vi "MagnetometerStateMachine-LakeshoreGaussMeter.vi"() -> ()   [LabVIEW 2014]
uses:
  <vilib>/MakerHub/LINX/Private/Local IO/LinxI2cWrite.vi
  <vilib>/MakerHub/LINX/Public/Utilities/Check Channel.vi
  <vilib>/MakerHub/LINX/Public/Utilities/Open Serial.vi
  <vilib>/MakerHub/LINX/Private/Utilties/Generate Error.vi
  <instrlib>/Stanford Research 830/Public/Data/Read (All Parameters).vi
  <vilib>/express/express shared/transition.llb/Dynamic To Waveform Array.vi
  <vilib>/express/express signal manip/GetorSetDDTAttributes/Get DDT Attributes/Get DDT Properties.xnode
  <vilib>/MakerHub/LINX/LMH-LINX.lvlib
  <instrlib>/Stanford Research 830/Stanford Research 830.lvlib
panel:
  out "data array":T1(array[cluster])
  in  "delta DAC":dbl=0.01 min=0.0 max=1.0 step=0.001 format="%#_13g"
  in  "max DAC":sgl=4.0 min=0 max=5 step=0.001
  in  "min DAC":dbl=1.0 min=0.0 max=5.0 step=0.001 format="%#_13g"
  out "Nloops2":i32
  out "Nloops":i32
  out "SRS-T":dbl
  out "SRS-R":dbl
  out "SRS-Y":dbl
  out "Parameter Values":T2
  out "XY Graph":T3(graph)
  out "SRS-X":dbl
  in  "Time Constant (8: 100ms)":u16(ring)=8 items=["10 us", "30 us", "100 us", "300 us", "1 ms", "3 ms", "10 ms", "30 ms", "100 ms", "300 ms", "1 s", "3 s", "10 s", "30 s", "100 s", "300 s", "1 ks", "3 ks", "10 ks", "30 ks"]
  in  "Internal Reference Frequency (1000 Hz)":dbl=20.0
  in  "Sine Output Amplitude (1 V)":dbl=1.0
  in  "Sensitivity (26: 1 V/uA)":i16(ring)=26 items=["Auto Gain"=-1, "2 nV/fA"=0, "5 nV/fA"=1, "10 nV/fA"=2, "20 nV/fA"=3, "50 nV/fA"=4, "100 nV/fA"=5, "200 nV/fA"=6, "500 nV/fA"=7, "1 uV/pA"=8, "2 uV/pA"=9, "5 uV/pA"=10, "10 uV/pA"=11, "20 uV/pA"=12, "50 uV/pA"=13, "100 uV/pA"=14, "200 uV/pA"=15, "500 uV/pA"=16, "1 mV/nA"=17, "2 mV/nA"=18, "5 mV/nA"=19, "10 mV/nA"=20, "20 mV/nA"=21, "50 mV/nA"=22, "100 mV/nA"=23, "200 mV/nA"=24, "500 mV/mA"=25, "1 V/uA"=26]
  in  "Dynamic Reserve (2: Low Noise)":i16(ring)=2 items=["High Reserve"=0, "Normal"=1, "Low Noise"=2, "Auto Reserve"=-1]
  in  "Reference Source (1: Internal)":u16(ring)=1 items=["External", "Internal"]
  in  "Input Coupling (0: AC)":u16(ring) items=["AC", "DC"]
  in  "Input Connection (0: Single-Ended Voltage)":u16(ring) items=["Single-Ended Voltage", "Differential Voltage", "1 MOhm Current Gain", "100 MOhm Current Gain"]
  in  "Current DAC Value":dbl
  in  "DAC Zeroing Voltage":dbl=2.5 min=0.0 max=5.0 step=0.001 format="%#_6f"
  out "Magnetic Field (Oe)":dbl
  in  "Choices":T4(ring)
  in  "End It All!":bool
  out "Error Out":errorcluster={"status"=FALSE, "code"=1073676294, "source"="VISA Read in LVH-LINX.lvlib:Device.lvlib:Serial Read.vi->LVH-LINX.lvlib:Device.lvlib:Wait For Packet.vi->LVH-LINX.lvlib:Device.lvlib:Send Command.vi->LVH-LINX.lvlib:Device.lvlib:Get DIO Channels.vi->LVH-LINX.lvlib:Device.lvlib:Load Device Config.vi->LVH-LINX.lvlib:Device.lvlib:Initialize Device.vi->LVH-LINX.lvlib:Initialize.vi->Untitled 2"}
  out "Device Name":string
  in  "Arduino Port":refnum<visa-resource-name>="N/A"
  # "Enter the voltage to get\nthe magnetic field to be zero."
  # "Input Signal"
  # "Reference"
  # "Sensitivity and Reserve"
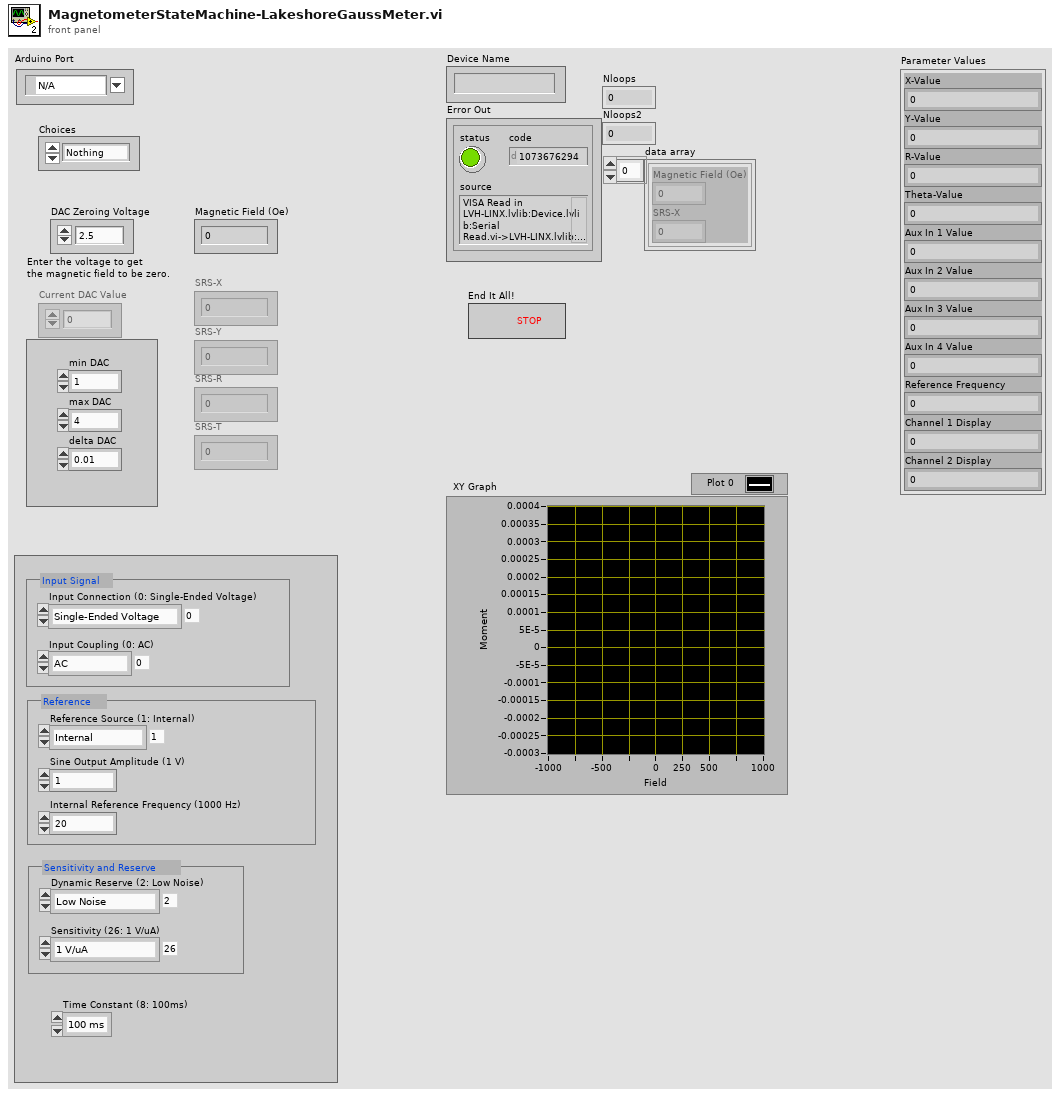
[diagram p1: front panel]
types:
  T1 = cluster{"Magnetic Field (Oe)":dbl, "SRS-X":dbl}[]
  T2 = cluster{"X-Value":dbl, "Y-Value":dbl, "R-Value":dbl, "Theta-Value":dbl, "Aux In 1 Value":dbl, "Aux In 2 Value":dbl, "Aux In 3 Value":dbl, "Aux In 4 Value":dbl, "Reference Frequency":dbl, "Channel 1 Display":dbl, "Channel 2 Display":dbl}
  T3 = cluster{"Magnetic Field (Oe)":dbl, "Moment":dbl}[]
  T4 = enum16{"Nothing", "Hysteresis", "MvsT", "SetTemperature", "ZeroHField"}
  T5 = typedef "LMH-LINX.lvlib/LINX Ref.ctl" = cluster{"IO":T6, "Interface":T7, "LINX Device Config":T8}
  T6 = typedef "LMH-LINX.lvlib/Platform.ctl" = enum16{"Remote", "Local"}
  T7 = typedef "LMH-LINX.lvlib/Interface.ctl" = enum16{"Serial", "TCP"}
  T8 = typedef "LMH-LINX.lvlib/Device.lvlib/LINX Device Config.ctl" = cluster{"Interface":T7, "COM Port":refnum<visa-resource-name>, "TCP Configuration":T9, "Device Family":u8, "Device ID":u8, "Device Name":string, "TCP Ref":refnum<k5>, "Channels":T10}
  T9 = typedef "LMH-LINX.lvlib/Device.lvlib/TCP Config.ctl" = cluster{"IP Address":string, "Port":u16}
  T10 = typedef "LMH-LINX.lvlib/Channels.ctl" = cluster{"DI":u8[], "DO":u8[], "AI":u8[], "AO":u8[], "PWM":u8[], "QE":u8[], "UART":u8[], "I2C 2":u8[], "SPI":u8[], "CAN":u8[], "Servo":u8[], "AI Ref (V)":dbl, "AI Resolution (Bits)":u8, "AO Ref (V)":dbl, "AO Resolution (Bits)":u8}
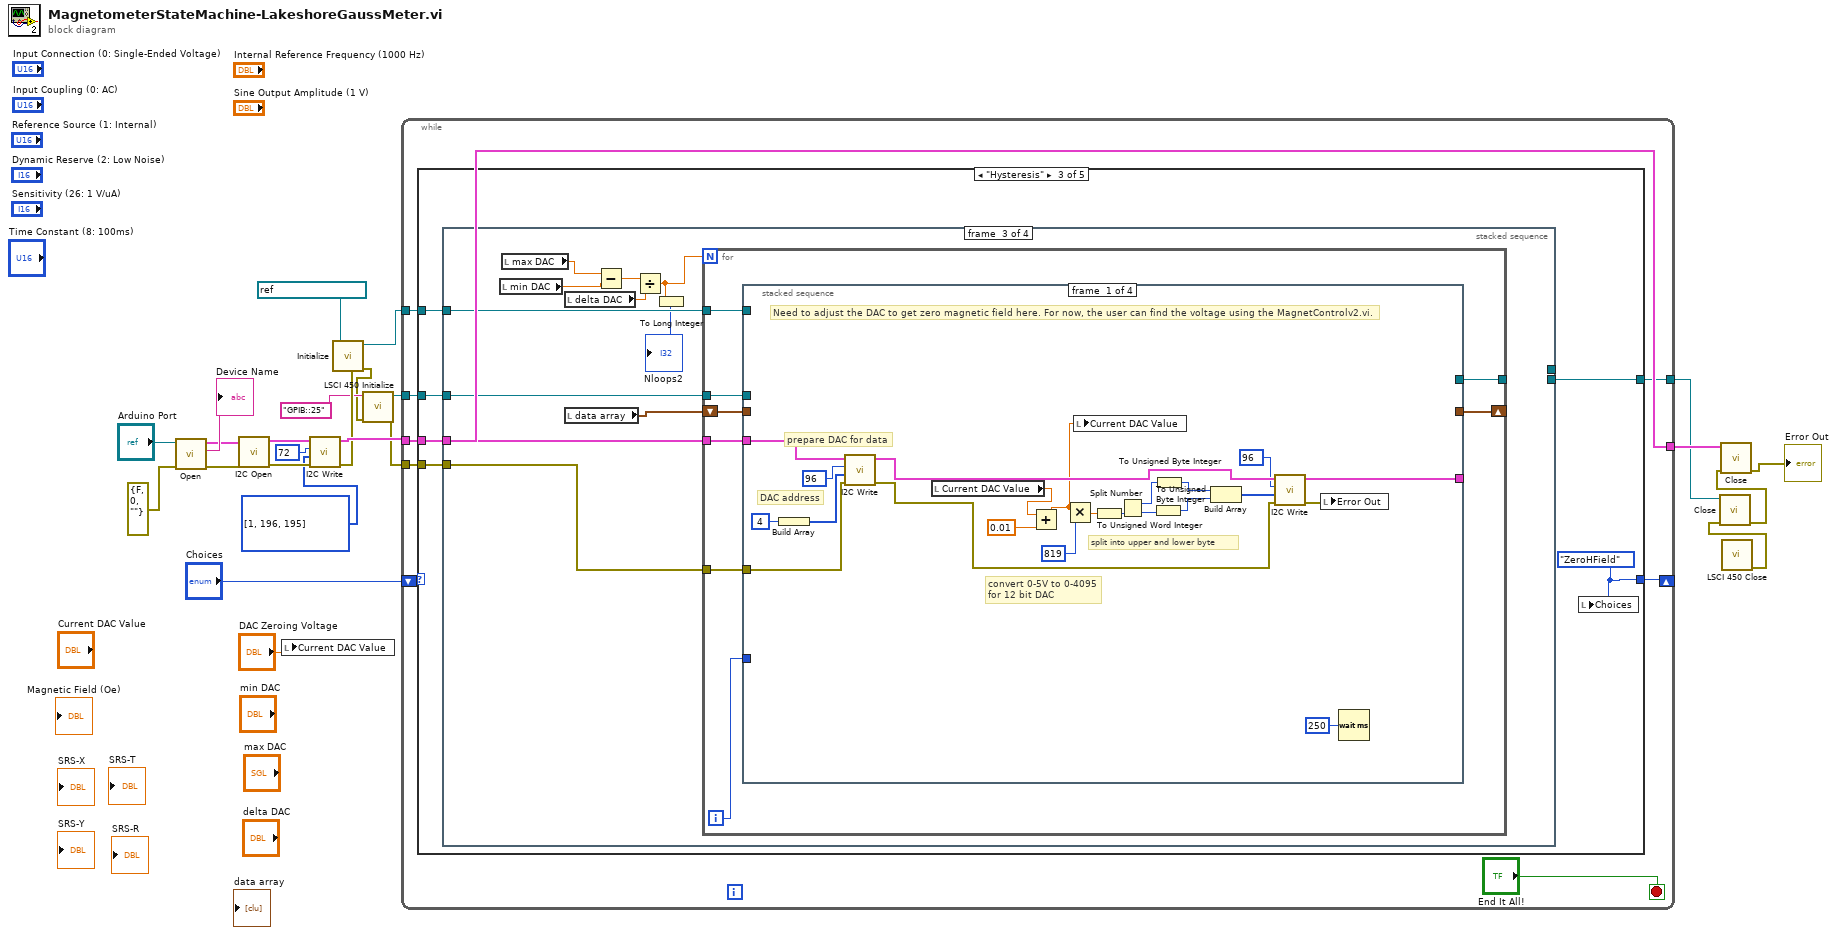
[diagram p0: block diagram]
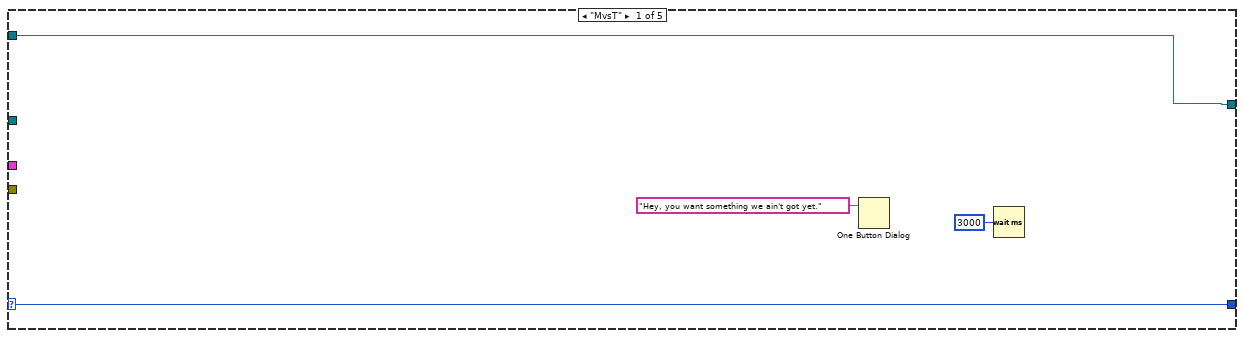
[diagram p2: hidden frame]
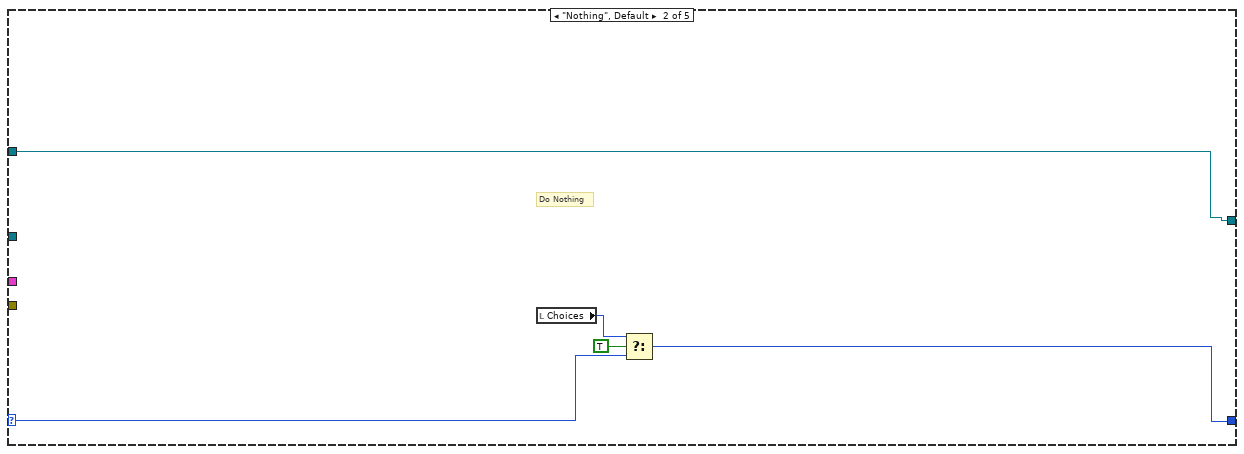
[diagram p3: hidden frame]
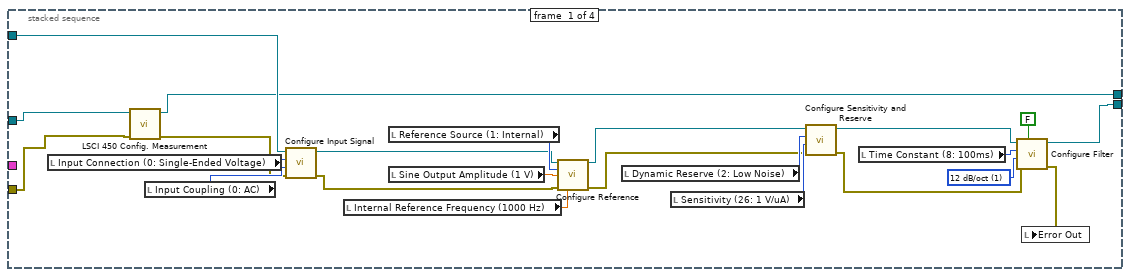
[diagram p4: hidden frame]
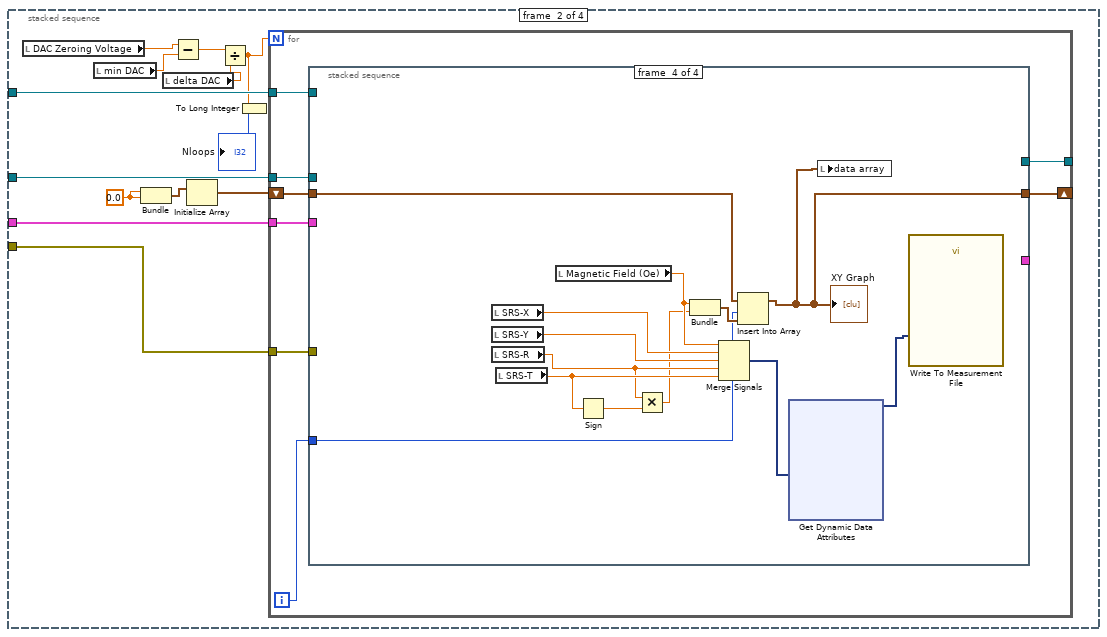
[diagram p5: hidden frame]
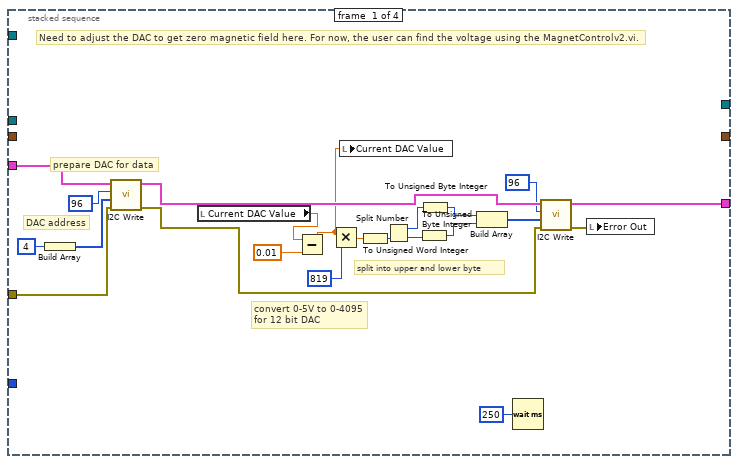
[diagram p6: hidden frame]
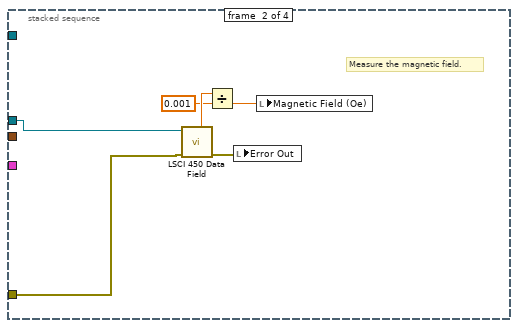
[diagram p7: hidden frame]
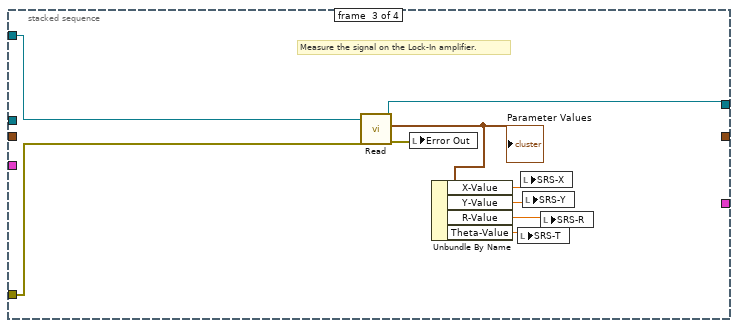
[diagram p8: hidden frame]
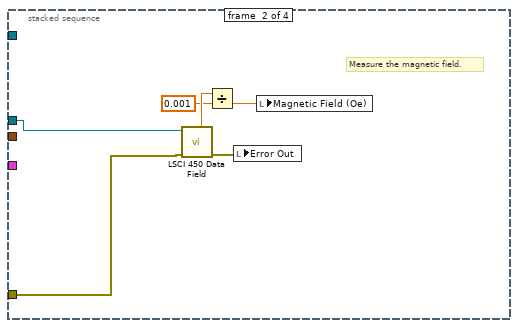
[diagram p9: hidden frame]
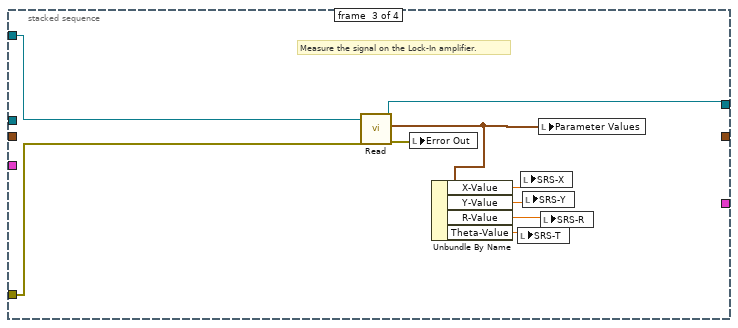
[diagram p10: hidden frame]
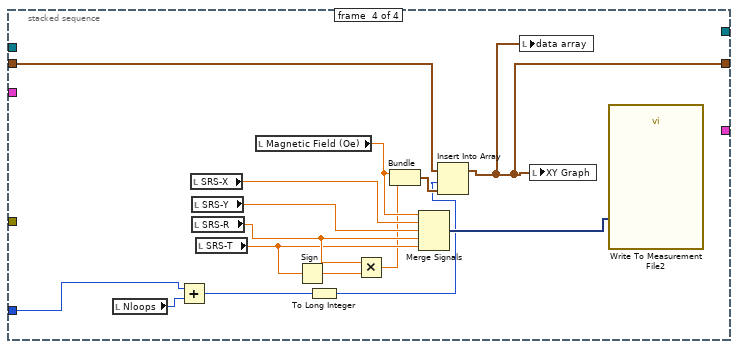
[diagram p11: hidden frame]
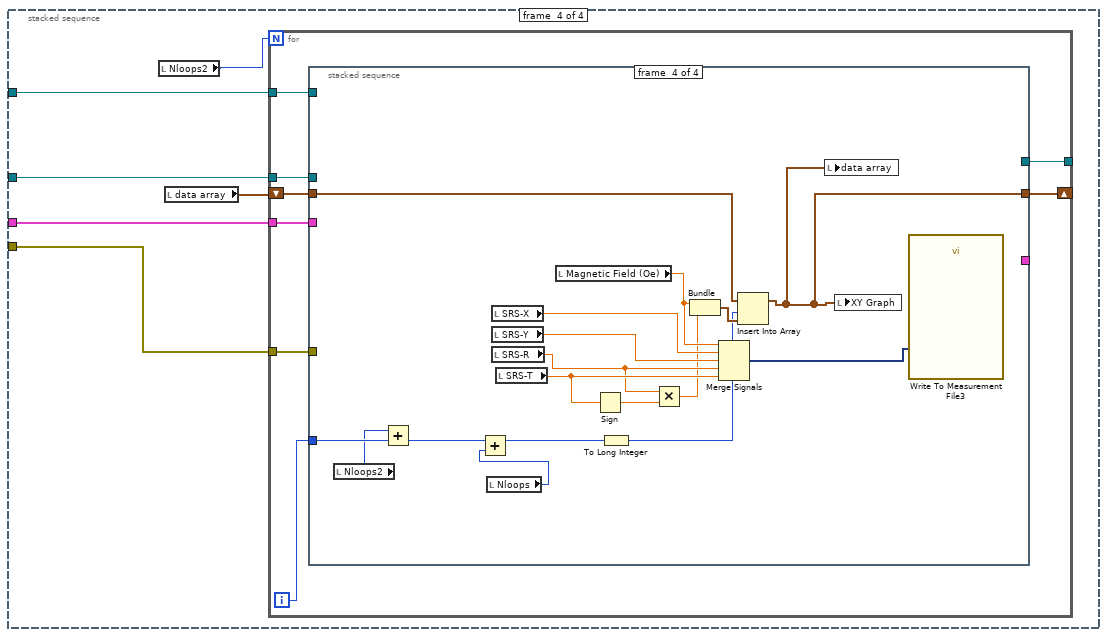
[diagram p12: hidden frame]
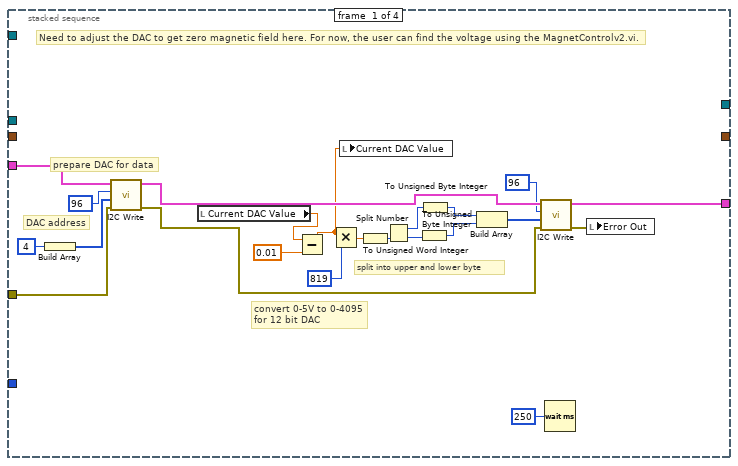
[diagram p13: hidden frame]
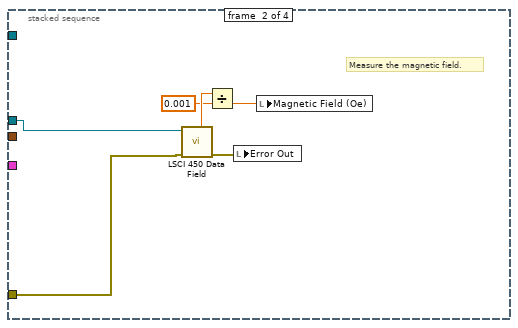
[diagram p14: hidden frame]
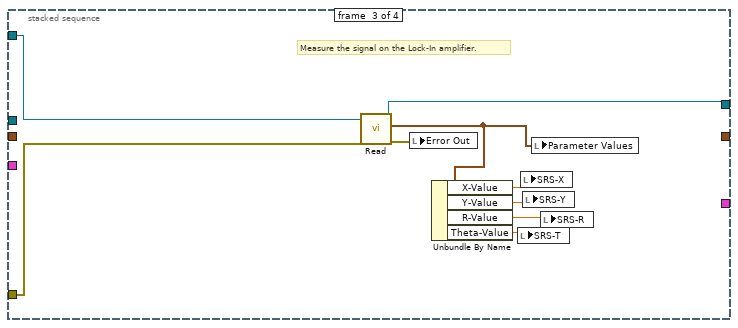
[diagram p15: hidden frame]
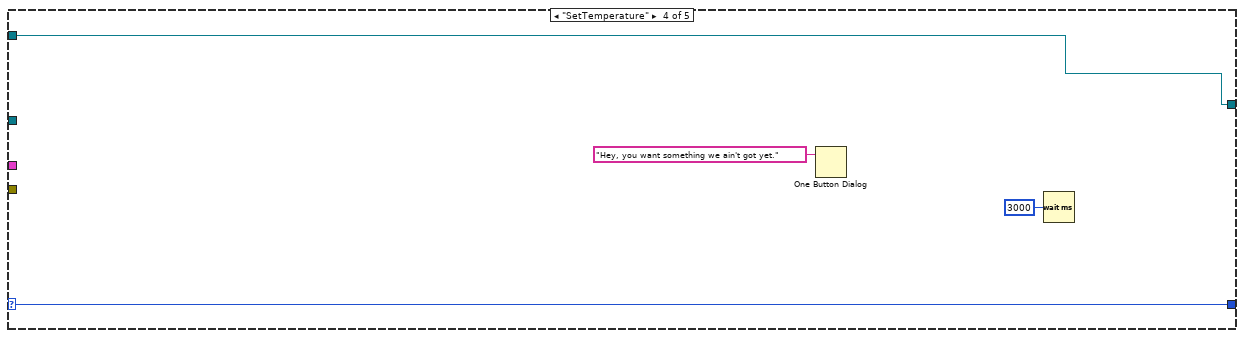
[diagram p16: hidden frame]
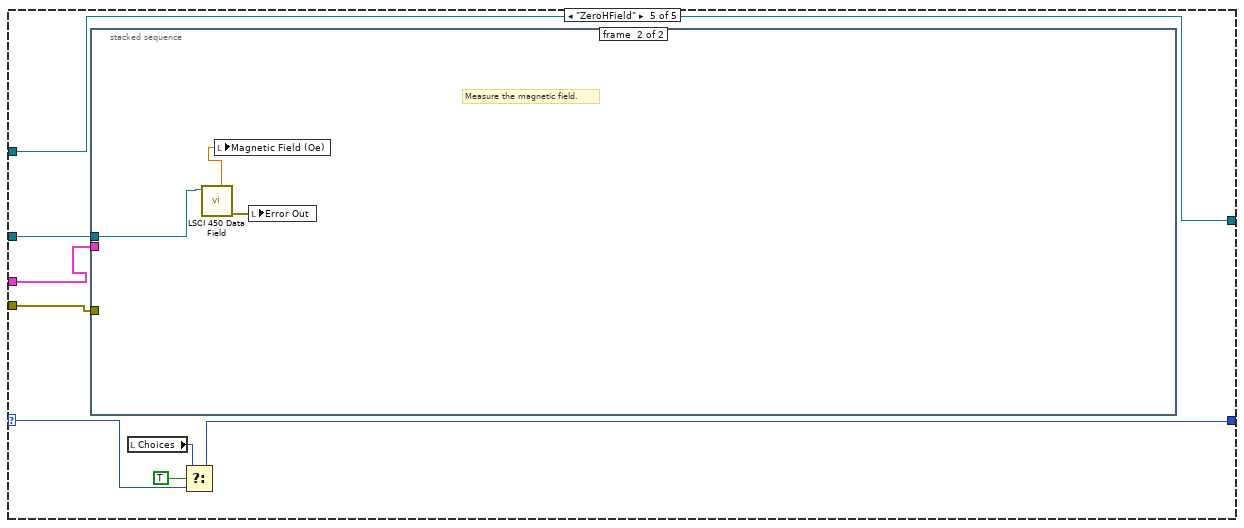
[diagram p17: hidden frame]
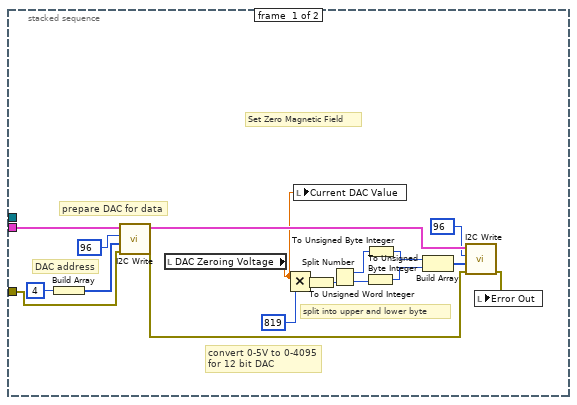
[diagram p18: hidden frame]
diagram:
  n1 = call-poly <vilib>:"Open.vi"("Error In"=errorcluster {"status"=FALSE, "code"=0, "source"=""}, "Serial Port"="Arduino Port") -> ("Error Out"=w19:errorcluster, "Device Name"=→"Device Name":string, "LINX Resource"=w20:T5)  [unwired: 7 in]
  n2 = call <vilib>:"I2C Open.vi"("Error In"=w19, "LINX Resource"=w20) -> ("Error Out"=w14:errorcluster, "LINX Resource"=w15:T5)  [unwired: 8 in]
  n3 = local write "Current DAC Value"("DAC Zeroing Voltage") -> ()
  n4 = call <vilib>:"I2C Write.vi"("Error In"=w14, "Data"=u8[] [1, 196, 195], "I2C Slave Address (0)"=u8 72, "LINX Resource"=w15) -> ("Error Out"=w9:errorcluster, "LINX Resource"=w16:T5)  [unwired: 6 in]
  n5 = call <instrlib>:"Initialize.vi"("error in (no error)"=w9, "VISA resource name"=refnum<visa-resource-name> "GPIB0::8::INSTR") -> ("error out"=w4:errorcluster, "VISA resource name out"=w8:refnum<visa-resource-name>)  [unwired: 8 in]
  n6 = call <instrlib>:"LSCI 450 Initialize.vi"("error in (no error)"=w4, "Instr. Descriptor (GPIB::12)"="GPIB::25" ("Gaussmeter (GPIB::25)")) -> ("error out"=w3:errorcluster, "VISA session"=w2:refnum<visa-resource-name>)  [unwired: 8 in]
  n7 = while {
    shift-right: [w29] -> _
    shift-left: "Choices" -> [w31]
    tunnel: w16 -> [w28]
    tunnel: w3 -> [w30]
    tunnel: [w28] -> w17
    tunnel: w8 -> [w27]
    tunnel: [w26] -> w7
    tunnel: w2 -> [w25]
    stop <- "End It All!" stop-if-true
    n8 = case shown="\"Hysteresis\"" w31 {
      selector: w31 -> [w35 w41 _ w292 w301]
      tunnel: w30 -> [_ _ w43 _ w300]
      tunnel: w28 -> [_ _ w47 _ w299]
      tunnel: [w35 w39 w46 w292 w298] -> w29
      tunnel: w27 -> [w33 w37 w45 w290 w295]
      tunnel: [w33 w37 w44 w290 w295] -> w26
      tunnel: w25 -> [_ _ w42 _ w294]
      frame "MvsT" {
        n9 = One Button Dialog(message="Hey, you want something we ain't got yet.") -> ()  [unwired: 1 in, 1 out]
        n10 = Wait (ms)(milliseconds to wait=u32 3000) -> ()  [unwired: 1 out]
      }
      frame "Nothing", Default {
        # "Do Nothing"
        n11 = local read "Choices"() -> (w40:T4)
        n12 = Select(t=w40, s=TRUE, f=w41) -> (s? t:f=w39:T4)
      }
      frame "Hysteresis" {
        w46 = T4."ZeroHField"
        n13 = stacked-sequence {
          tunnel: w47 -> [_ w83 w161 w227]
          tunnel: w45 -> [w61 w82 w160 w226]
          tunnel: [w57 _ _ _] -> w44
          tunnel: w43 -> [w49 w81 w159 w225]
          tunnel: w42 -> [w51 w80 w158 w224]
          tunnel: [w50 _ _ _] -> _
          frame #0 {
            w63 = u16 1 items=["6 dB/oct", "12 dB/oct", "18 db/oct", "24 dB/oct"] ("Low Pass Filter Slope (1: 12dB/oct)")
            n14 = local read "Input Connection (0: Single-Ended Voltage)"() -> (w70:u16)
            n15 = call <instrlib>:"LSCI 450 Config. Measurement.vi"("error in (no error)"=w49, "VISA session"=w51) -> ("error out"=w48:errorcluster, "dup VISA session"=w50:refnum<visa-resource-name>)  [unwired: 8 in]
            n16 = local read "Input Coupling (0: AC)"() -> (w69:u16)
            n17 = call <instrlib>:"Configure Input Signal.vi"("error in (no error)"=w48, "Input Coupling (0: AC)"=w69, "Input Connection (0: Single-Ended Voltage)"=w70, "VISA resource name"=w61) -> ("error out"=w56:errorcluster, "VISA resource name out"=w60:refnum<visa-resource-name>)  [unwired: 6 in]
            n18 = local read "Internal Reference Frequency (1000 Hz)"() -> (w66:dbl)
            n19 = local read "Reference Source (1: Internal)"() -> (w67:u16)
            n20 = local read "Sine Output Amplitude (1 V)"() -> (w68:dbl)
            n21 = call <instrlib>:"Configure Reference.vi"("VISA resource name"=w60, "Reference Source (1: Internal)"=w67, "Sine Output Amplitude (1 V)"=w68, "error in (no error)"=w56, "Internal Reference Frequency (1000 Hz)"=w66) -> ("VISA resource name out"=w59:refnum<visa-resource-name>, "error out"=w55:errorcluster)  [unwired: 9 in]
            n22 = local read "Dynamic Reserve (2: Low Noise)"() -> (w64:i16)
            n23 = local read "Sensitivity (26: 1 V/uA)"() -> (w65:i16)
            n24 = call <instrlib>:"Configure Sensitivity and Reserve.vi"("error in (no error)"=w55, "Sensitivity (-1: Auto gain)"=w65, "Dynamic Reserve (-1: Auto Reserve)"=w64, "VISA resource name"=w59) -> ("error out"=w54:errorcluster, "VISA resource name out"=w58:refnum<visa-resource-name>)  [unwired: 6 in]
            n25 = local read "Time Constant (8: 100ms)"() -> (w62:u16)
            n26 = call <instrlib>:"Configure Filter.vi"("Enable Sync Filter (F: Disable)"=FALSE, "error in (no error)"=w54, "Low Pass Filter Slope (1: 12dB/oct)"=w63, "Time Constant (8: 100ms)"=w62, "VISA resource name"=w58) -> ("error out"=w52:errorcluster, "VISA resource name out"=w57:refnum<visa-resource-name>)  [unwired: 5 in]
            n27 = local write "Error Out"(w52) -> ()
          }
          frame #1 {
            w71 = 0.0
            n28 = local read "DAC Zeroing Voltage"() -> (w78:dbl)
            n29 = local read "min DAC"() -> (w76:dbl)
            n30 = Bundle(w71, w71) -> (w72:cluster{dbl, dbl})  [unwired: 1 in]
            n31 = local read "delta DAC"() -> (w75:dbl)
            n32 = Subtract(x=w78, y=w76) -> (x-y=w77:dbl)
            n33 = Initialize Array(w72) -> (w73:cluster{dbl, dbl}[])  [unwired: 1 in]
            n34 = Divide(x=w77, y=w75) -> (x/y=w79:dbl)
            n35 = To Long Integer(number=w79) -> (32bit integer=→"Nloops":i32)
            n36 = for {
              N: w79 -> [_]
              tunnel: w81 -> [w90]
              tunnel: w83 -> [w91]
              tunnel: w82 -> [w89]
              tunnel: [w88] -> _
              shift-right: [w87] -> _
              shift-left: w73 -> [w86]
              tunnel: w80 -> [w85]
              i -> [w84]
              n37 = stacked-sequence {
                tunnel: [w113 _ _ _] -> _
                tunnel: w91 -> [w112 _ _ _]
                tunnel: w90 -> [w106 w118 w126 _]
                tunnel: w89 -> [_ _ w127 _]
                tunnel: w84 -> [_ _ _ w140]
                tunnel: [_ _ w125 _] -> w88
                tunnel: [_ _ _ w135] -> w87
                tunnel: w86 -> [_ _ _ w139]
                tunnel: w85 -> [_ w119 _ _]
                frame #0 {
                  # "convert 0-5V to 0-4095\nfor 12 bit DAC"
                  # "split into upper and lower byte"
                  # "Need to adjust the DAC to get zero magnetic field here. For now, the user can find the voltage using the MagnetControlv2.vi."
                  # "DAC address"
                  # "prepare DAC for data"
                  n38 = Build Array(u8 4) -> (w107:u8[])
                  n39 = call <vilib>:"I2C Write.vi"("Error In"=w106, "Data"=w107, "I2C Slave Address (0)"=u8 96, "LINX Resource"=w112) -> ("Error Out"=w110:errorcluster, "LINX Resource"=w109:T5)  [unwired: 6 in]
                  n40 = local read "Current DAC Value"() -> (w95:dbl)
                  n41 = Subtract(x=w95, y=0.01) -> (x-y=w93:dbl)
                  n42 = Multiply(x=w93, y=u32 819) -> (x*y=w97:dbl)
                  n43 = local write "Current DAC Value"(w93) -> ()
                  n44 = To Unsigned Word Integer(number=w97) -> (unsigned 16bit integer=w99:u16)
                  n45 = Split Number(x=w99) -> (hi(x)=w100:u8, lo(x)=w104:u8)
                  n46 = To Unsigned Byte Integer(number=w104) -> (unsigned 8bit integer=w102:u8)
                  n47 = To Unsigned Byte Integer(number=w100) -> (unsigned 8bit integer=w103:u8)
                  n48 = Build Array(w103, w102) -> (w101:u8[])
                  n49 = Wait (ms)(milliseconds to wait=u32 250) -> ()  [unwired: 1 out]
                  n50 = call <vilib>:"I2C Write.vi"("Error In"=w110, "Data"=w101, "I2C Slave Address (0)"=u8 96, "LINX Resource"=w109) -> ("Error Out"=w96:errorcluster, "LINX Resource"=w113:T5)  [unwired: 6 in]
                  n51 = local write "Error Out"(w96) -> ()
                }
                frame #1 {
                  # "Measure the magnetic field."
                  n52 = call <instrlib>:"LSCI 450 Data Field.vi"("error in (no error)"=w118, "VISA session"=w119) -> ("error out"=w117:errorcluster, "Field (0.00)"=w115:dbl)  [unwired: 5 in, 3 out]
                  n53 = Divide(x=w115, y=0.001) -> (x/y=w116:dbl)
                  n54 = local write "Error Out"(w117) -> ()
                  n55 = local write "Magnetic Field (Oe)"(w116) -> ()
                }
                frame #2 {
                  # "Measure the signal on the Lock-In amplifier."
                  n56 = call-poly <instrlib>:"Read.vi"("error in (no error)"=w126, "VISA resource name"=w127) -> ("error out"=w128:errorcluster, "Parameter Values"=w124:T2, "VISA resource name out"=w125:refnum<visa-resource-name>)  [unwired: 7 in]
                  "Parameter Values" <- w124
                  n57 = local write "Error Out"(w128) -> ()
                  n58 = Unbundle By Name(w124) -> ("X-Value"=w122:dbl, "Y-Value"=w120:dbl, "R-Value"=w123:dbl, "Theta-Value"=w121:dbl)
                  n59 = local write "SRS-T"(w121) -> ()
                  n60 = local write "SRS-X"(w122) -> ()
                  n61 = local write "SRS-Y"(w120) -> ()
                  n62 = local write "SRS-R"(w123) -> ()
                }
                frame #3 {
                  n63 = local read "SRS-X"() -> (w137:dbl)
                  n64 = local read "SRS-Y"() -> (w136:dbl)
                  n65 = local read "SRS-R"() -> (w130:dbl)
                  n66 = local read "SRS-T"() -> (w132:dbl)
                  n67 = local read "Magnetic Field (Oe)"() -> (w138:dbl)
                  n68 = Sign(1:w132) -> (0:w131:dbl)
                  n69 = Multiply(x=w130, y=w131) -> (x*y=w129:dbl)
                  n70 = Bundle("Magnetic Field (Oe)"=w138, w129) -> (w141:cluster{"Magnetic Field (Oe)":dbl, dbl})  [unwired: 1 in]
                  n71 = Merge Signals(w138, w137, w136, w130, w132) -> (w134:dynamicdata)
                  n72 = Insert Into Array(array=w139, index=w140, new element=w141) -> (w135:cluster{dbl, dbl}[])
                  "XY Graph" <- w135
                  n73 = xnode "Get Dynamic Data Attributes"("Signals In"=w134) -> ("Signals Out"=w133:dynamicdata)  [unwired: 2 in, 2 out]
                  n74 = local write "data array"(w135) -> ()
                  n75 = call "Write To Measurement File"("Signals"=w133) -> ()  [unwired: 16 in, 3 out]
                }
              }
            }
          }
          frame #2 {
            n76 = local read "min DAC"() -> (w155:dbl)
            n77 = local read "max DAC"() -> (w154:sgl)
            n78 = local read "delta DAC"() -> (w153:dbl)
            n79 = local read "data array"() -> (w152:T1)
            n80 = Subtract(x=w154, y=w155) -> (x-y=w157:dbl)
            n81 = Divide(x=w157, y=w153) -> (x/y=w156:dbl)
            n82 = To Long Integer(number=w156) -> (32bit integer=→"Nloops2":i32)
            n83 = for {
              N: w156 -> [_]
              tunnel: w159 -> [w168]
              tunnel: w161 -> [w169]
              tunnel: w160 -> [w167]
              tunnel: [w166] -> _
              shift-right: [w165] -> _
              shift-left: w152 -> [w164]
              tunnel: w158 -> [w163]
              i -> [w162]
              n84 = stacked-sequence {
                tunnel: [w191 _ _ _] -> _
                tunnel: w169 -> [w190 _ _ _]
                tunnel: w168 -> [w184 w196 w204 _]
                tunnel: w167 -> [_ _ w205 _]
                tunnel: w162 -> [_ _ _ w215]
                tunnel: [_ _ w203 _] -> w166
                tunnel: [_ _ _ w211] -> w165
                tunnel: w164 -> [_ _ _ w220]
                tunnel: w163 -> [_ w197 _ _]
                frame #0 {
                  # "convert 0-5V to 0-4095\nfor 12 bit DAC"
                  # "split into upper and lower byte"
                  # "Need to adjust the DAC to get zero magnetic field here. For now, the user can find the voltage using the MagnetControlv2.vi."
                  # "DAC address"
                  # "prepare DAC for data"
                  n85 = Build Array(u8 4) -> (w185:u8[])
                  n86 = call <vilib>:"I2C Write.vi"("Error In"=w184, "Data"=w185, "I2C Slave Address (0)"=u8 96, "LINX Resource"=w190) -> ("Error Out"=w188:errorcluster, "LINX Resource"=w187:T5)  [unwired: 6 in]
                  n87 = local read "Current DAC Value"() -> (w173:dbl)
                  n88 = Add(x=w173, y=0.01) -> (x+y=w171:dbl)
                  n89 = Multiply(x=w171, y=u32 819) -> (x*y=w175:dbl)
                  n90 = local write "Current DAC Value"(w171) -> ()
                  n91 = To Unsigned Word Integer(number=w175) -> (unsigned 16bit integer=w177:u16)
                  n92 = Split Number(x=w177) -> (hi(x)=w178:u8, lo(x)=w182:u8)
                  n93 = To Unsigned Byte Integer(number=w182) -> (unsigned 8bit integer=w180:u8)
                  n94 = To Unsigned Byte Integer(number=w178) -> (unsigned 8bit integer=w181:u8)
                  n95 = Build Array(w181, w180) -> (w179:u8[])
                  n96 = call <vilib>:"I2C Write.vi"("Error In"=w188, "Data"=w179, "I2C Slave Address (0)"=u8 96, "LINX Resource"=w187) -> ("Error Out"=w174:errorcluster, "LINX Resource"=w191:T5)  [unwired: 6 in]
                  n97 = local write "Error Out"(w174) -> ()
                  n98 = Wait (ms)(milliseconds to wait=u32 250) -> ()  [unwired: 1 out]
                }
                frame #1 {
                  # "Measure the magnetic field."
                  n99 = call <instrlib>:"LSCI 450 Data Field.vi"("error in (no error)"=w196, "VISA session"=w197) -> ("error out"=w195:errorcluster, "Field (0.00)"=w193:dbl)  [unwired: 5 in, 3 out]
                  n100 = Divide(x=w193, y=0.001) -> (x/y=w194:dbl)
                  n101 = local write "Error Out"(w195) -> ()
                  n102 = local write "Magnetic Field (Oe)"(w194) -> ()
                }
                frame #2 {
                  # "Measure the signal on the Lock-In amplifier."
                  n103 = call-poly <instrlib>:"Read.vi"("error in (no error)"=w204, "VISA resource name"=w205) -> ("error out"=w206:errorcluster, "Parameter Values"=w198:T2, "VISA resource name out"=w203:refnum<visa-resource-name>)  [unwired: 7 in]
                  n104 = local write "Error Out"(w206) -> ()
                  n105 = Unbundle By Name(w198) -> ("X-Value"=w201:dbl, "Y-Value"=w199:dbl, "R-Value"=w202:dbl, "Theta-Value"=w200:dbl)
                  n106 = local write "SRS-T"(w200) -> ()
                  n107 = local write "SRS-X"(w201) -> ()
                  n108 = local write "SRS-Y"(w199) -> ()
                  n109 = local write "Parameter Values"(w198) -> ()
                  n110 = local write "SRS-R"(w202) -> ()
                }
                frame #3 {
                  n111 = local read "Nloops"() -> (w214:i32)
                  n112 = Add(x=w215, y=w214) -> (x+y=w213:i32)
                  n113 = local read "SRS-X"() -> (w217:dbl)
                  n114 = local read "SRS-Y"() -> (w216:dbl)
                  n115 = local read "SRS-R"() -> (w210:dbl)
                  n116 = local read "SRS-T"() -> (w209:dbl)
                  n117 = local read "Magnetic Field (Oe)"() -> (w219:dbl)
                  n118 = Sign(1:w209) -> (0:w208:dbl)
                  n119 = To Long Integer(number=w213) -> (32bit integer=w212:i32)
                  n120 = Multiply(x=w210, y=w208) -> (x*y=w207:dbl)
                  n121 = Bundle("Magnetic Field (Oe)"=w219, w207) -> (w221:cluster{"Magnetic Field (Oe)":dbl, dbl})  [unwired: 1 in]
                  n122 = Merge Signals(w219, w217, w216, w210, w209) -> (w218:dynamicdata)
                  n123 = Insert Into Array(array=w220, index=w212, new element=w221) -> (w211:T1)
                  n124 = local write "data array"(w211) -> ()
                  n125 = local write "XY Graph"(w211) -> ()
                  n126 = call "Write To Measurement File2"("Signals"=w218) -> ()  [unwired: 16 in, 3 out]
                }
              }
            }
          }
          frame #3 {
            n127 = local read "Nloops2"() -> (w222:i32)
            n128 = local read "data array"() -> (w223:T1)
            n129 = for {
              N: w222 -> [_]
              tunnel: w225 -> [w234]
              tunnel: w227 -> [w235]
              tunnel: w226 -> [w233]
              tunnel: [w232] -> _
              shift-right: [w231] -> _
              shift-left: w223 -> [w230]
              tunnel: w224 -> [w229]
              i -> [w228]
              n130 = stacked-sequence {
                tunnel: [w257 _ _ _] -> _
                tunnel: w235 -> [w256 _ _ _]
                tunnel: w234 -> [w250 w262 w270 _]
                tunnel: w233 -> [_ _ w271 _]
                tunnel: w228 -> [_ _ _ w288]
                tunnel: [_ _ w269 _] -> w232
                tunnel: [_ _ _ w277] -> w231
                tunnel: w230 -> [_ _ _ w287]
                tunnel: w229 -> [_ w263 _ _]
                frame #0 {
                  # "convert 0-5V to 0-4095\nfor 12 bit DAC"
                  # "split into upper and lower byte"
                  # "Need to adjust the DAC to get zero magnetic field here. For now, the user can find the voltage using the MagnetControlv2.vi."
                  # "DAC address"
                  # "prepare DAC for data"
                  n131 = Build Array(u8 4) -> (w251:u8[])
                  n132 = call <vilib>:"I2C Write.vi"("Error In"=w250, "Data"=w251, "I2C Slave Address (0)"=u8 96, "LINX Resource"=w256) -> ("Error Out"=w254:errorcluster, "LINX Resource"=w253:T5)  [unwired: 6 in]
                  n133 = local read "Current DAC Value"() -> (w239:dbl)
                  n134 = Subtract(x=w239, y=0.01) -> (x-y=w237:dbl)
                  n135 = Multiply(x=w237, y=u32 819) -> (x*y=w241:dbl)
                  n136 = local write "Current DAC Value"(w237) -> ()
                  n137 = To Unsigned Word Integer(number=w241) -> (unsigned 16bit integer=w243:u16)
                  n138 = Split Number(x=w243) -> (hi(x)=w244:u8, lo(x)=w248:u8)
                  n139 = To Unsigned Byte Integer(number=w248) -> (unsigned 8bit integer=w246:u8)
                  n140 = To Unsigned Byte Integer(number=w244) -> (unsigned 8bit integer=w247:u8)
                  n141 = Build Array(w247, w246) -> (w245:u8[])
                  n142 = call <vilib>:"I2C Write.vi"("Error In"=w254, "Data"=w245, "I2C Slave Address (0)"=u8 96, "LINX Resource"=w253) -> ("Error Out"=w240:errorcluster, "LINX Resource"=w257:T5)  [unwired: 6 in]
                  n143 = Wait (ms)(milliseconds to wait=u32 250) -> ()  [unwired: 1 out]
                  n144 = local write "Error Out"(w240) -> ()
                }
                frame #1 {
                  # "Measure the magnetic field."
                  n145 = call <instrlib>:"LSCI 450 Data Field.vi"("error in (no error)"=w262, "VISA session"=w263) -> ("error out"=w261:errorcluster, "Field (0.00)"=w259:dbl)  [unwired: 5 in, 3 out]
                  n146 = Divide(x=w259, y=0.001) -> (x/y=w260:dbl)
                  n147 = local write "Error Out"(w261) -> ()
                  n148 = local write "Magnetic Field (Oe)"(w260) -> ()
                }
                frame #2 {
                  # "Measure the signal on the Lock-In amplifier."
                  n149 = call-poly <instrlib>:"Read.vi"("error in (no error)"=w270, "VISA resource name"=w271) -> ("error out"=w272:errorcluster, "Parameter Values"=w264:T2, "VISA resource name out"=w269:refnum<visa-resource-name>)  [unwired: 7 in]
                  n150 = local write "Error Out"(w272) -> ()
                  n151 = Unbundle By Name(w264) -> ("X-Value"=w267:dbl, "Y-Value"=w265:dbl, "R-Value"=w268:dbl, "Theta-Value"=w266:dbl)
                  n152 = local write "SRS-T"(w266) -> ()
                  n153 = local write "SRS-X"(w267) -> ()
                  n154 = local write "SRS-Y"(w265) -> ()
                  n155 = local write "Parameter Values"(w264) -> ()
                  n156 = local write "SRS-R"(w268) -> ()
                }
                frame #3 {
                  n157 = local read "Nloops2"() -> (w281:i32)
                  n158 = Add(x=w281, y=w288) -> (x+y=w282:i32)
                  n159 = local read "Nloops"() -> (w279:i32)
                  n160 = Add(x=w282, y=w279) -> (x+y=w280:i32)
                  n161 = local read "SRS-X"() -> (w284:dbl)
                  n162 = local read "SRS-Y"() -> (w283:dbl)
                  n163 = local read "SRS-R"() -> (w274:dbl)
                  n164 = local read "SRS-T"() -> (w276:dbl)
                  n165 = local read "Magnetic Field (Oe)"() -> (w286:dbl)
                  n166 = Sign(1:w276) -> (0:w275:dbl)
                  n167 = To Long Integer(number=w280) -> (32bit integer=w278:i32)
                  n168 = Multiply(x=w274, y=w275) -> (x*y=w273:dbl)
                  n169 = Bundle("Magnetic Field (Oe)"=w286, w273) -> (w289:cluster{"Magnetic Field (Oe)":dbl, dbl})  [unwired: 1 in]
                  n170 = Merge Signals(w286, w284, w283, w274, w276) -> (w285:dynamicdata)
                  n171 = Insert Into Array(array=w287, index=w278, new element=w289) -> (w277:T1)
                  n172 = local write "data array"(w277) -> ()
                  n173 = local write "XY Graph"(w277) -> ()
                  n174 = call "Write To Measurement File3"("Signals"=w285) -> ()  [unwired: 16 in, 3 out]
                }
              }
            }
          }
        }
        n175 = local write "Choices"(w46) -> ()
      }
      frame "SetTemperature" {
        n176 = One Button Dialog(message="Hey, you want something we ain't got yet.") -> ()  [unwired: 1 in, 1 out]
        n177 = Wait (ms)(milliseconds to wait=u32 3000) -> ()  [unwired: 1 out]
      }
      frame "ZeroHField" {
        n178 = stacked-sequence {
          tunnel: w300 -> [w305 _]
          tunnel: w299 -> [w303 _]
          tunnel: w294 -> [_ w322]
          frame #0 {
            # "convert 0-5V to 0-4095\nfor 12 bit DAC"
            # "split into upper and lower byte"
            # "DAC address"
            # "prepare DAC for data"
            # "Set Zero Magnetic Field"
            n179 = Build Array(u8 4) -> (w315:u8[])
            n180 = call <vilib>:"I2C Write.vi"("Error In"=w305, "Data"=w315, "I2C Slave Address (0)"=u8 96, "LINX Resource"=w303) -> ("Error Out"=w318:errorcluster, "LINX Resource"=w317:T5)  [unwired: 6 in]
            n181 = local read "DAC Zeroing Voltage"() -> (w304:dbl)
            n182 = Multiply(x=w304, y=u32 819) -> (x*y=w306:dbl)
            n183 = local write "Current DAC Value"(w304) -> ()
            n184 = To Unsigned Word Integer(number=w306) -> (unsigned 16bit integer=w308:u16)
            n185 = Split Number(x=w308) -> (hi(x)=w309:u8, lo(x)=w313:u8)
            n186 = To Unsigned Byte Integer(number=w313) -> (unsigned 8bit integer=w311:u8)
            n187 = To Unsigned Byte Integer(number=w309) -> (unsigned 8bit integer=w312:u8)
            n188 = Build Array(w312, w311) -> (w310:u8[])
            n189 = call <vilib>:"I2C Write.vi"("Error In"=w318, "Data"=w310, "I2C Slave Address (0)"=u8 96, "LINX Resource"=w317) -> ("Error Out"=w302:errorcluster)  [unwired: 6 in, 1 out]
            n190 = local write "Error Out"(w302) -> ()
          }
          frame #1 {
            # "Measure the magnetic field."
            n191 = call <instrlib>:"LSCI 450 Data Field.vi"("VISA session"=w322) -> ("error out"=w320:errorcluster, "Field (0.00)"=w321:dbl)  [unwired: 6 in, 3 out]
            n192 = local write "Magnetic Field (Oe)"(w321) -> ()
            n193 = local write "Error Out"(w320) -> ()
          }
        }
        n194 = local read "Choices"() -> (w297:T4)
        n195 = Select(t=w297, s=TRUE, f=w301) -> (s? t:f=w298:T4)
      }
    }
  }
  n196 = call <instrlib>:"LSCI 450 Close.vi"() -> ("error out"=w1:errorcluster)  [unwired: 11 in]
  n197 = call <vilib>:"Close.vi"("error in (no error)"=w1, "VISA resource name"=w7) -> ("error out"=w6:errorcluster)  [unwired: 9 in]
  n198 = call <vilib>:"Close.vi"("Error In"=w6, "LINX Resource"=w17) -> ("Error Out"=→"Error Out":errorcluster)  [unwired: 9 in]
